vi "CC Convert RA and DEC to HHMMSS.vi"(11 "RA and DEC":T3) -> (0 "DEC String":string, 1 "RA String":string, 2 "Declination":T1 {"Arc Sec" format="%0#2_6g"}, 3 "Right Ascension":T2)   [LabVIEW 2021]
uses:
  typedefs/CC cluster RA and DEC.ctl
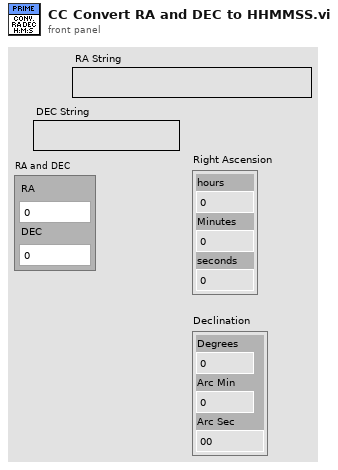
[diagram p1: front panel]
types:
  T1 = cluster{"Degrees":dbl, "Arc Min":dbl, "Arc Sec":dbl}
  T2 = cluster{"hours":dbl, "Minutes":dbl, "seconds":dbl}
  T3 = typedef "CC cluster RA and DEC.ctl" = cluster{"RA":dbl, "DEC":dbl}
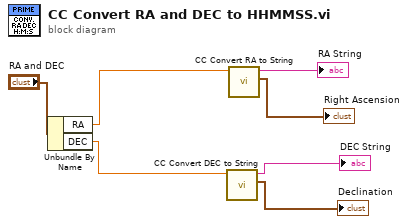
[diagram p0: block diagram]
diagram:
  n1 = Unbundle By Name("RA and DEC") -> ("RA"=w3:dbl, "DEC"=w6:dbl)
  n2 = call "CC Convert DEC to String.vi"("DEC"=w6) -> ("Declination"=→"Declination":T1, "DEC String"=→"DEC String":string)  [unwired: 8 in, 1 out]
  n3 = call "CC Convert RA to String.vi"("RA"=w3) -> ("Right Ascension"=→"Right Ascension":T2, "RA String"=→"RA String":string)  [unwired: 8 in, 1 out]
